vi "GetCtlRef_Core.vi"(8 "error in (no error)":errorcluster, 10 "CtlName In":string, 11 "ctlRef_Maps in":refnum<class "ctlRef_Maps.lvclass">) -> (0 "error out":errorcluster, 1 "Ctl Refnum":refnum<vi>, 2 "CtlName out":string, 3 "ctlRef_Maps out":refnum<class "ctlRef_Maps.lvclass">, 4 "Found":bool)   [LabVIEW 2020, in "CtlReferences.lvlib" / "ctlRef_Maps.lvclass"]
uses:
  ctlRef_Maps.lvclass
  ctlRef_Maps.lvclass/ctlRef_Maps.ctl
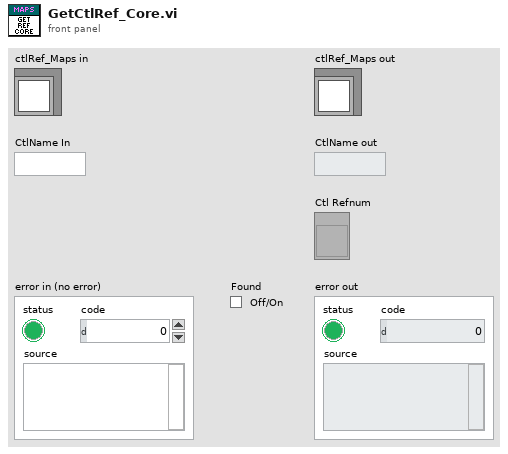
[diagram p1: front panel]
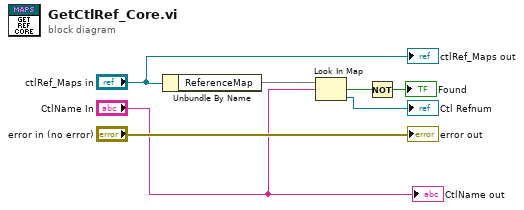
[diagram p0: block diagram]
diagram:
  n1 = Unbundle By Name("ctlRef_Maps in") -> ("ReferenceMap"=w5:map{string, refnum<vi>})
  n2 = Look In Map(map=w5, key="CtlName In") -> (key not found?=w2:bool, value=→"Ctl Refnum":refnum<vi>)  [unwired: 1 in]
  n3 = Not(x=w2) -> (.not. x?=→"Found":bool)
  "CtlName out" <- "CtlName In"
  "ctlRef_Maps out" <- "ctlRef_Maps in"
  "error out" <- "error in (no error)"
